vi "New Edit Element.vi"(8 "error in (no error)":errorcluster, 11 "Product-A in":refnum<class "Product-A.lvclass">) -> (0 "error out":errorcluster, 3 "Product-A out":refnum<class "Product-A.lvclass">)   [LabVIEW 2018, in "Product-A.lvclass"]
uses:
  Product-A.lvclass
  U:/modules/labview-orm/_Serializable Base Object/_ISerializable.lvclass
  U:/modules/labview-orm/demo/Product.lvclass
  <vilib>/Utility/error.llb/Error Cluster From Error Code.vi
  <vilib>/ErrorRing/Error Ring.xnode
panel:
  in  "owner":string
  in  "display name":string
  out "uid":u64
  in  "numeric":i64
  in  "isObsolete":bool
  in  "status":u8
  in  "project name":string
  in  "cancel button":bool
  in  "ok button":bool
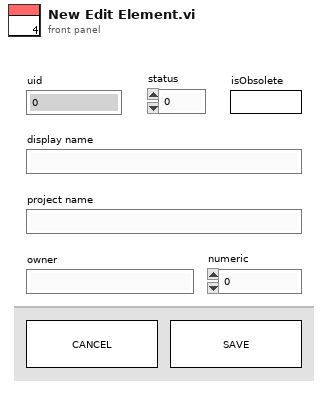
[diagram p1: front panel]
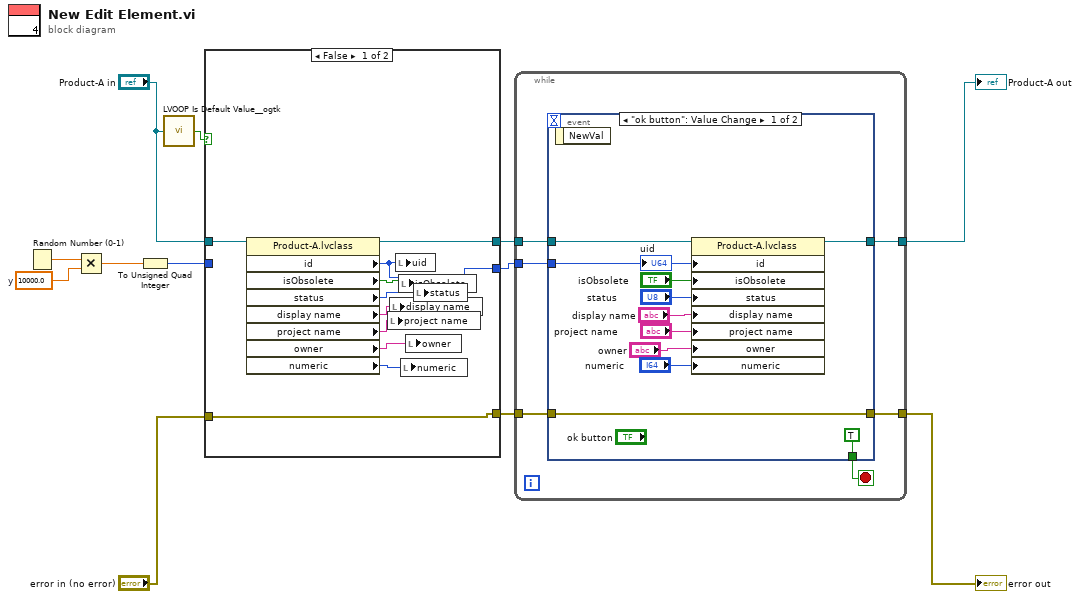
[diagram p0: block diagram]
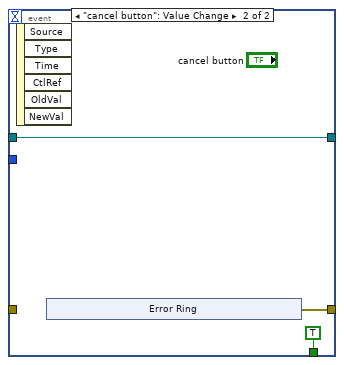
[diagram p3: hidden frame]
diagram:
  w11 = 10000.0  # y
  n1 = Random Number (0-1)() -> (number: 0 to 1=w12:dbl)
  n2 = Multiply(x=w12, y=w11) -> (x*y=w10:dbl)
  n3 = To Unsigned Quad Integer(1:w10) -> (0:w2:u64)
  n4 = call <userlib>:"LVOOP Is Default Value__ogtk.vi"("Object"="Product-A in") -> ("Is Default Value?"=w3:bool)
  n5 = case shown="False" w3 {
    tunnel: "Product-A in" -> [w22 w23]
    tunnel: [w21 w23] -> w7
    tunnel: [w20 w25] -> w6
    tunnel: "error in (no error)" -> [w20 w25]
    tunnel: w2 -> [_ w24]
    tunnel: [w19 w24] -> w1
    frame False {
      n6 = property class="Product-A.lvclass"(reference=w22) -> (reference out=w21:refnum<class "Product-A.lvclass">, "id"=w19:i32, "isObsolete"=w13:bool, "status"=w14:u8, "display name"=w15:string, "project name"=w16:string, "owner"=w17:string, "numeric"=w18:i64)  [unwired: 1 in, 1 out]
      n7 = local write "project name"(w16) -> ()
      n8 = local write "display name"(w15) -> ()
      n9 = local write "uid"(w19) -> ()
      n10 = local write "isObsolete"(w13) -> ()
      n11 = local write "numeric"(w18) -> ()
      n12 = local write "owner"(w17) -> ()
      n13 = local write "status"(w14) -> ()
    }
    frame True {
    }
  }
  n14 = while {
    tunnel: w6 -> [w28]
    tunnel: w7 -> [w31]
    tunnel: [w30] -> w8
    tunnel: [w29] -> w9
    tunnel: w1 -> [w26]
    stop <- w27 stop-if-true
    n15 = event shown="[0] \"ok button\": Value Change" {
      selector: _ -> [_ _]
      dyn-events: _ -> [_ _]
      timeout: _ -> [_ _]
      tunnel: w31 -> [w42 w45]
      tunnel: [w41 w45] -> w30
      tunnel: [w40 w44] -> w29
      tunnel: w28 -> [w40 _]
      tunnel: [TRUE TRUE] -> w27
      tunnel: w26 -> [w38 _]
      event "ok button": Value Change {
        n16 = event-data() -> ()  [unwired: 1 in, 1 out]
        n17 = property class="Product-A.lvclass"(reference=w42, "id"=w38, "isObsolete"="isObsolete", "status"="status", "display name"="display name", "project name"="project name", "owner"="owner", "numeric"="numeric") -> (reference out=w41:refnum<class "Product-A.lvclass">)  [unwired: 1 in, 1 out]
        "uid" <- w38
      }
      event "cancel button": Value Change {
        n18 = event-data() -> ()  [unwired: 1 in, 6 out]
        n19 = xnode "Error Ring"() -> ("error out"=w44:errorcluster)
      }
    }
  }
  "error out" <- w9
  "Product-A out" <- w8
